vi "Pass.vi"(7 "Caller":string, 8 "error in (no error)":errorcluster, 10 "Assertion":string, 11 "Test Framework in":refnum<class "Test Framework.lvclass">) -> (0 "error out":errorcluster, 3 "Test Framework out":refnum<class "Test Framework.lvclass">)   [LabVIEW 2017, in "Transparent Assertions.lvlib" / "Test Framework.lvclass"]
doc: "Executes the unit test framework-specific operation to indicate a passing test."
uses:
  Test Framework.lvclass
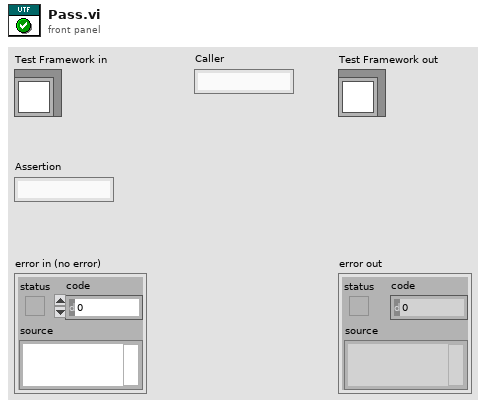
[diagram p1: front panel]
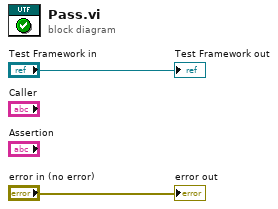
[diagram p0: block diagram]
diagram:
  "error out" <- "error in (no error)"
  "Test Framework out" <- "Test Framework in"
